vi "sub_LF_set_slit.vi"(8 "error in (no error)":errorcluster, 10 "Numeric In":dbl, 11 "LightField Automation in":refnum<class "LightField Automation.lvclass">) -> (0 "error out":errorcluster, 2 "Numeric Out":dbl, 3 "LightField Automation out":refnum<class "LightField Automation.lvclass">)   [LabVIEW 2015]
uses:
  Ligth Field/lightfield-automation-labview/LightField Automation.lvclass
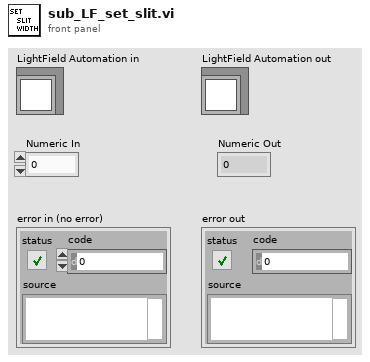
[diagram p1: front panel]
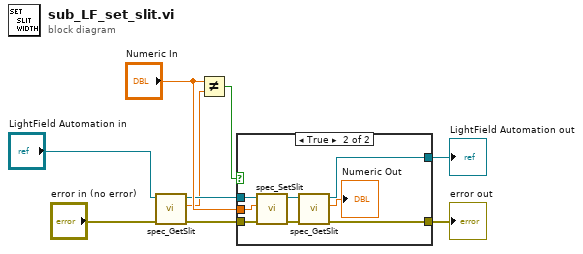
[diagram p0: block diagram]
diagram:
  n1 = call "spec_GetSlit.vi"("error in (no error)"="error in (no error)", "LightField Automation in"="LightField Automation in") -> ("error out"=w2:errorcluster, "Slit Width"=w1:dbl, "LightField Automation out"=w4:refnum<class "LightField Automation.lvclass">)  [unwired: 7 in]
  n2 = Not Equal?(x="Numeric In", y=w1) -> (x != y?=w7:bool)
  n3 = case shown="True" w7 {
    tunnel: "Numeric In" -> [_ w18]
    tunnel: [w11 w13] -> w8
    tunnel: [w10 w12] -> w9
    tunnel: w4 -> [w11 w19]
    tunnel: w2 -> [w10 w17]
    frame False {
    }
    frame True {
      n4 = call "spec_SetSlit.vi"("error in (no error)"=w17, "WidthSelected"=w18, "LightField Automation in"=w19) -> ("error out"=w15:errorcluster, "LightField Automation out"=w16:refnum<class "LightField Automation.lvclass">)  [unwired: 7 in]
      n5 = call "spec_GetSlit.vi"("error in (no error)"=w15, "LightField Automation in"=w16) -> ("error out"=w12:errorcluster, "Slit Width"=→"Numeric Out":dbl, "LightField Automation out"=w13:refnum<class "LightField Automation.lvclass">)  [unwired: 7 in]
    }
  }
  "error out" <- w9
  "LightField Automation out" <- w8
